vi "ParseArgumentsCore.vi"(8 "error in (no error)":errorcluster, 9 "Value":string, 10 "Option":string, 11 "ExecuteMultipleBuildSpecs in":refnum<class "ExecuteMultipleBuildSpecs.lvclass">) -> (0 "error out":errorcluster, 3 "ExecuteMultipleBuildSpecs out":refnum<class "ExecuteMultipleBuildSpecs.lvclass">)   [LabVIEW 2020, in "ExecuteMultipleBuildSpecs.lvclass"]
doc: "VI to be overridden by child classes to parse operation-specific arguments."
uses:
  ExecuteMultipleBuildSpecs.lvclass
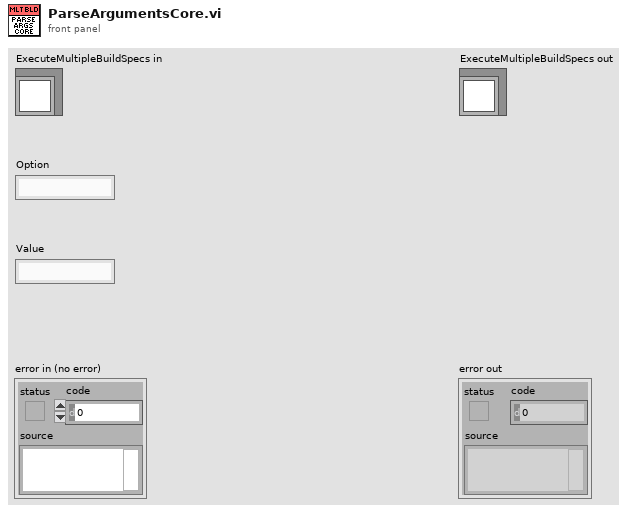
[diagram p1: front panel]
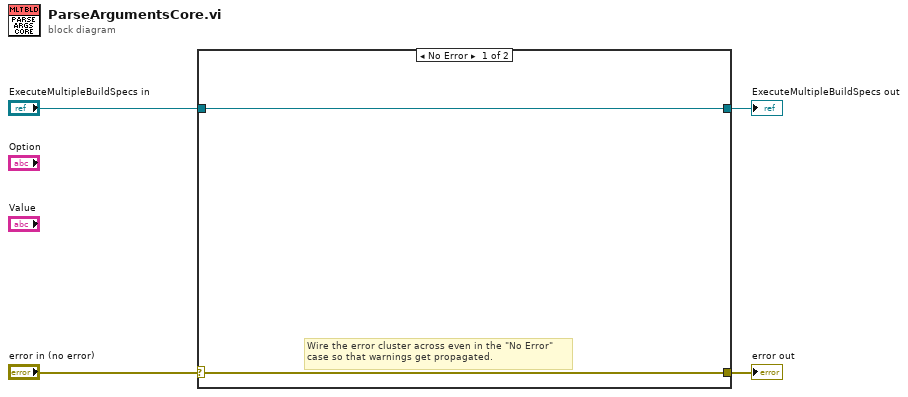
[diagram p0: block diagram]
diagram:
  n1 = case shown="No Error" "error in (no error)" {
    selector: "error in (no error)" -> [w5 w8]
    tunnel: [w5 w8] -> w3
    tunnel: [w6 w7] -> w1
    tunnel: "ExecuteMultipleBuildSpecs in" -> [w6 w7]
    frame No Error {
      # "Wire the error cluster across even in the \"No Error\"\ncase so that warnings get propagated."
    }
    frame Error {
    }
  }
  "error out" <- w3
  "ExecuteMultipleBuildSpecs out" <- w1
